vi "(SubVI) Create offset array.vi"(9 "Frame #":u32, 10 "pixel# of a image":i32, 11 "Frame# of one .Glimpse \n(2Gb)":u32) -> (3 "Array":cluster{"offset":T1, u32}[](array[cluster]))   [LabVIEW 2014]
uses:
  4.Other/header ctl/Offset.ctl
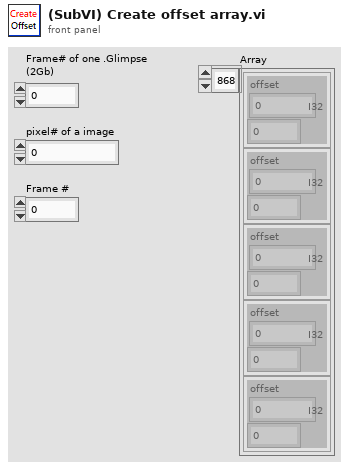
[diagram p1: front panel]
types:
  T1 = typedef "Offset.ctl" = i32
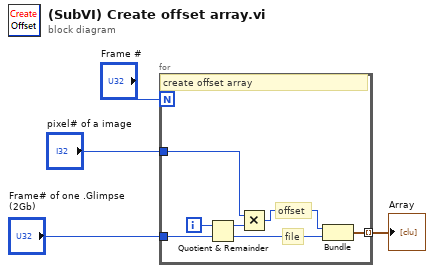
[diagram p0: block diagram]
diagram:
  n1 = for {
    N: "Frame #" -> [_]
    tunnel: "pixel# of a image" -> [w7]
    tunnel: [w11] -> w4 mode=indexing
    tunnel: "Frame# of one .Glimpse \n(2Gb)" -> [w9]
    i -> [w8]
    # "offset"
    # "file"
    # "create offset array"
    n2 = Quotient & Remainder(x=w8, y=w9) -> (x-y*floor(x/y)=w6:u32, floor(x/y)=w5:u32)
    n3 = Multiply(x=w7, y=w6) -> (x*y=w10:u32)
    n4 = Bundle(w10, w5) -> (w11:cluster{u32, u32})  [unwired: 1 in]
  }
  "Array" <- w4
